vi "JSON GENERADOR.vi"(8 "error in":errorcluster, 9 "Boolean":bool, 10 "Value":refnum<class "JSON Value.lvclass">, 11 "JSON Object in":refnum<class "JSON Object.lvclass">) -> (0 "error out":errorcluster, 3 "JSON Object out":refnum<class "JSON Object.lvclass">)   [LabVIEW 2015]
uses:
  <vilib>/addons/JSON API/Get Polymorphic/JSON GetSet.lvlib
  <vilib>/addons/JSON API/JSON Object/Set Object Item by name.vi
  <vilib>/addons/JSON API/JSON Object/JSON Object.lvclass
  <vilib>/addons/JSON API/JSON Value/JSON Value.lvclass
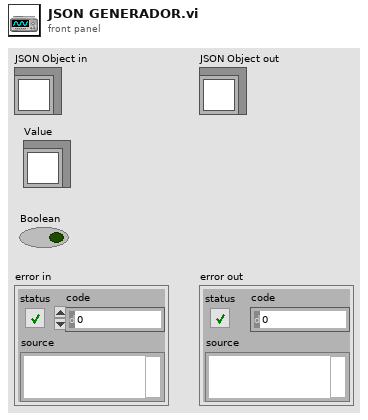
[diagram p1: front panel]
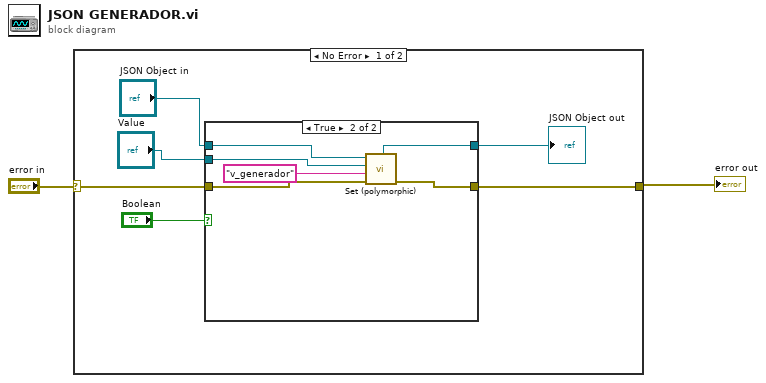
[diagram p0: block diagram]
diagram:
  n1 = case shown="No Error" "error in" {
    selector: "error in" -> [w4 w17]
    tunnel: [w5 w17] -> w1
    frame No Error {
      n2 = case shown="True" "Boolean" {
        tunnel: "JSON Object in" -> [w10 w15]
        tunnel: w4 -> [w9 w14]
        tunnel: [w10 w13] -> w7
        tunnel: [w9 w12] -> w5
        tunnel: "Value" -> [_ w11]
        frame False {
        }
        frame True {
          n3 = call-poly <vilib>:"Set (polymorphic).vi"("error in (no error)"=w14, "name"="v_generador", "Value"=w11, "JSON Object in"=w15) -> ("error out"=w12:errorcluster, "JSON Object out"=w13:refnum<class "JSON Object.lvclass">)  [unwired: 5 in, 1 out]
        }
      }
      "JSON Object out" <- w7
    }
    frame Error {
    }
  }
  "error out" <- w1
